vi "Write Active Bus.vi"(8 "error in (no error)":errorcluster, 10 "ActBus":u32, 11 "DigitalGraph.lvclass in":refnum<class "DigitalGraph.lvclass">) -> (0 "error out":errorcluster, 3 "DigitalGraph.lvclass out":refnum<class "DigitalGraph.lvclass">)   [LabVIEW 2015, in "DigitalGraph.lvclass"]
uses:
  DigitalGraph.lvclass
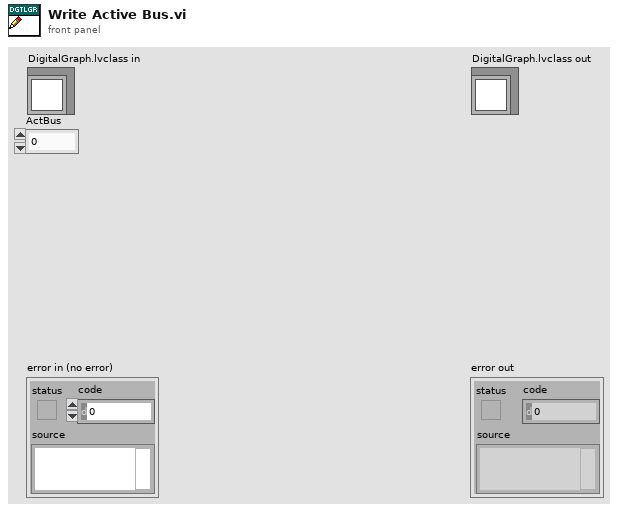
[diagram p1: front panel]
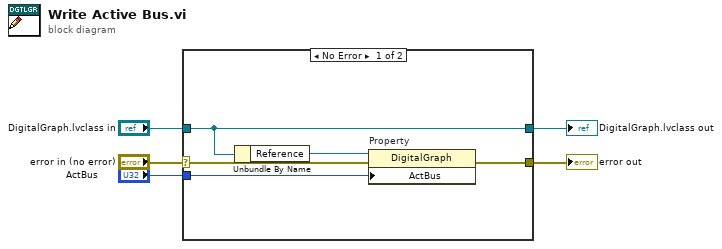
[diagram p0: block diagram]
diagram:
  n1 = case shown="No Error" "error in (no error)" {
    selector: "error in (no error)" -> [w6 w12]
    tunnel: [w10 w12] -> w4
    tunnel: [w8 w11] -> w2
    tunnel: "DigitalGraph.lvclass in" -> [w8 w11]
    tunnel: "ActBus" -> [w9 _]
    frame No Error {
      n2 = Unbundle By Name(w8) -> ("Reference"=w7:refnum<vi>)
      n3 = property on="Property" class="DigitalGraph"(reference=w7, error in=w6, "ActBus"=w9) -> (error out=w10:errorcluster)  [unwired: 1 out]
    }
    frame Error {
    }
  }
  "error out" <- w4
  "DigitalGraph.lvclass out" <- w2
